vi "AP2_cold_head_control.vi"() -> ()   [LabVIEW 2023]
panel:
  in  "Tab Control":enum32{"Controls", "Monitoring"}(tab)
  in  "stop":bool
  in  "Master Control":bool
  in  "Cold Head Auto Start Time":timestamp format="%<%H:%M:%S>T"
  in  "Target Temperature / K":dbl=4.5 min=4.5 max=500.0 step=1.0
  out "Current Temperature / K":dbl
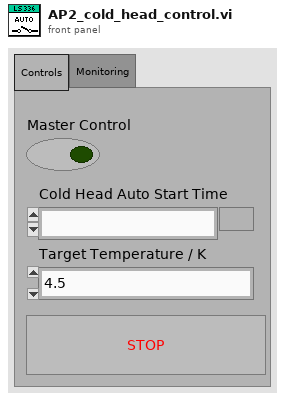
[diagram p1: front panel]
types:
  T1 = cluster{"second":i32, "minute":i32, "hour":i32, "day of month":i32, "month":i32, "year":i32, "day of week":i32, "day of year":i32, "is DST":i32}
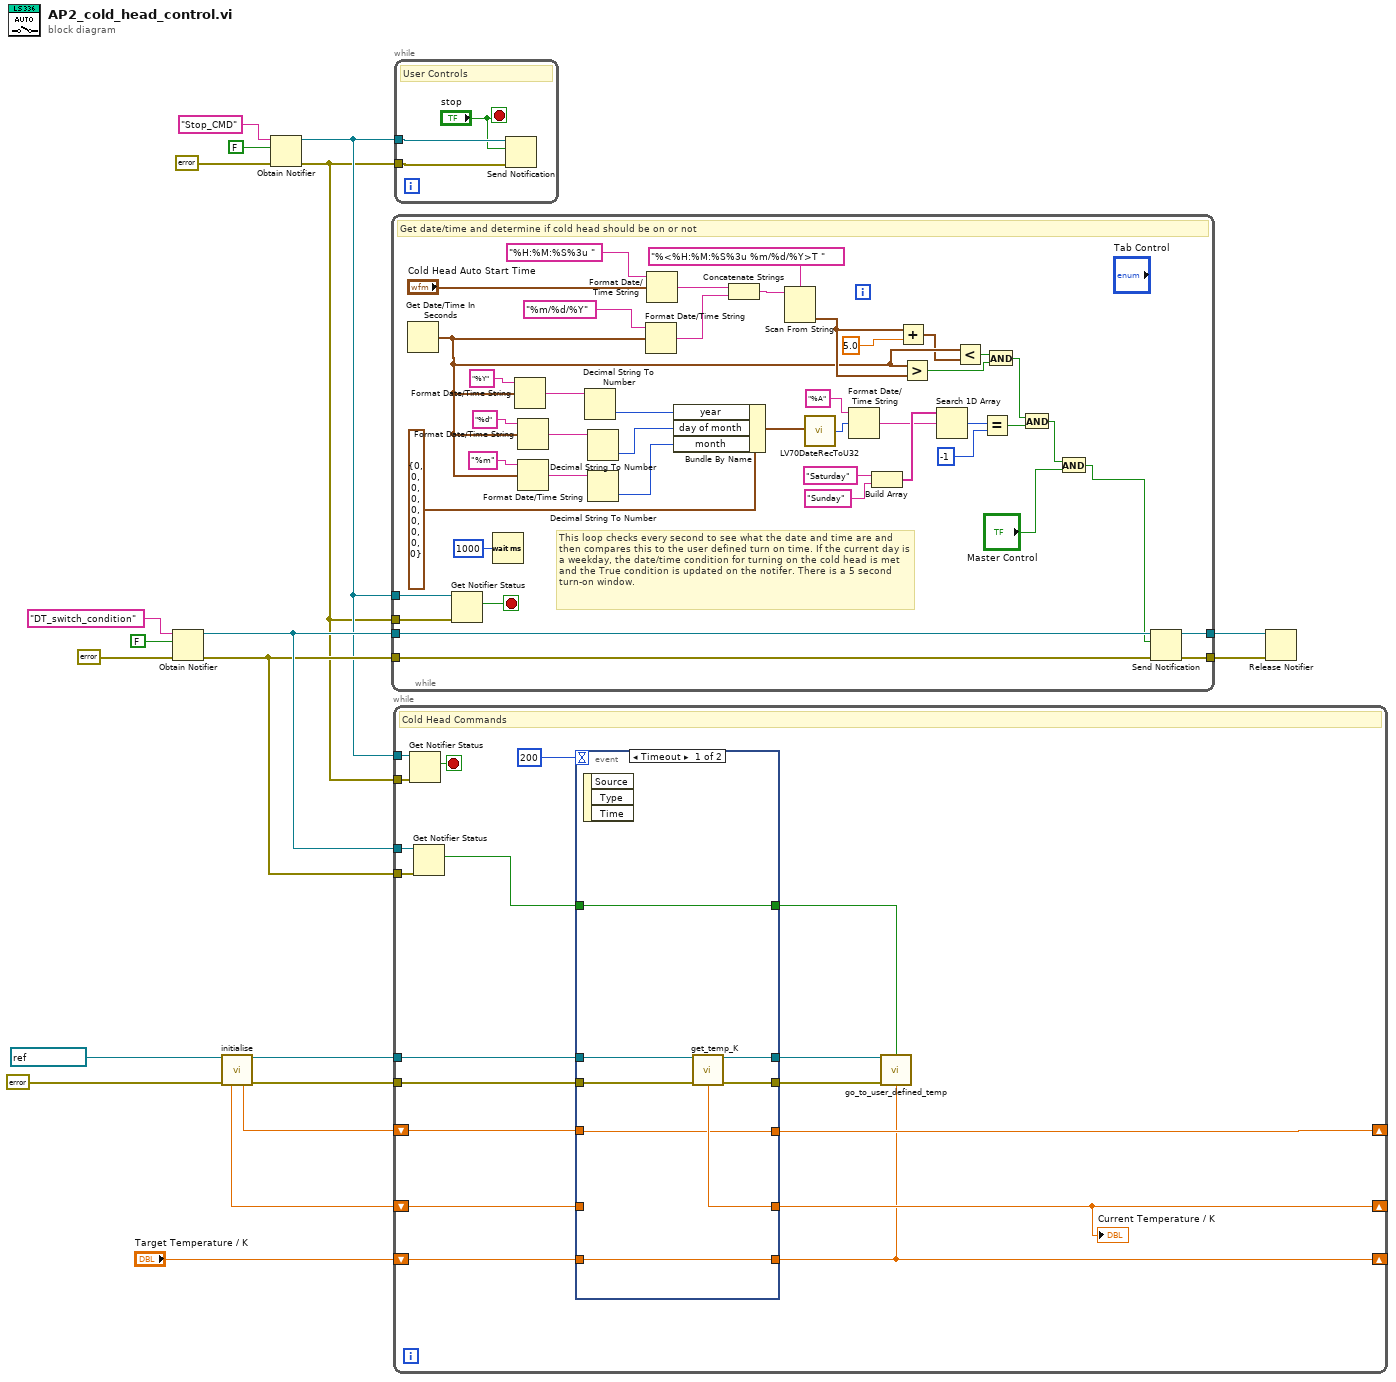
[diagram p0: block diagram]
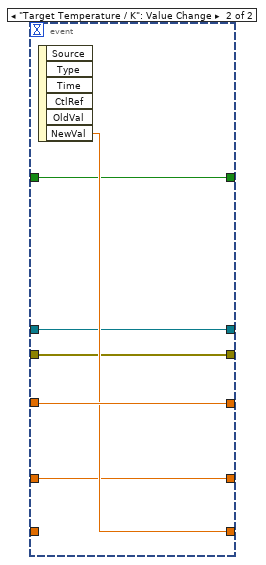
[diagram p2: hidden frame]
diagram:
  n1 = Obtain Notifier(name (unnamed)="DT_switch_condition", notification data type=FALSE, error in (no error)=errorcluster {"status"=FALSE, "code"=0, "source"=""}) -> (notifier out=w14:refnum<notifier>, error out=w13:errorcluster)  [unwired: 1 in, 1 out]
  n2 = call "initialise.vi"("VISA resource name"=refnum<visa-resource-name> "CH_Cntrl", "error in (no error)"=errorcluster {"status"=FALSE, "code"=0, "source"=""}) -> ("VISA resource name out"=w4:refnum<visa-resource-name>, "Cold Head Temperature / K"=w2:dbl, "Current Setpoint / K"=w1:dbl, "error out"=w3:errorcluster)  [unwired: 10 in]
  n3 = Obtain Notifier(name (unnamed)="Stop_CMD", notification data type=FALSE, error in (no error)=errorcluster {"status"=FALSE, "code"=0, "source"=""}) -> (notifier out=w9:refnum<notifier>, error out=w8:errorcluster)  [unwired: 1 in, 1 out]
  n4 = while {
    tunnel: w14 -> [w36]
    tunnel: w13 -> [w35]
    tunnel: [w34] -> w16
    tunnel: [w33] -> w15
    tunnel: w9 -> [w32]
    tunnel: w8 -> [w31]
    stop <- w30 stop-if-true
    # "This loop checks every second to see what the date and time are and then compares this to the user defined turn on time. If the current day is a weekday, the date/time condition for turning on the cold head is met and the True condition is updated on the notifer. There is a 5 second turn-on window."
    # "Get date/time and determine if cold head should be on or not"
    n5 = Get Date/Time In Seconds() -> (seconds since 1Jan1904=w24:timestamp)
    n6 = Get Notifier Status(notifier=w32, error in (no error)=w31) -> (current notification=w30:bool)  [unwired: 4 out]
    n7 = Wait (ms)(milliseconds to wait=u32 1000) -> ()  [unwired: 1 out]
    n8 = Format Date/Time String(time format string (%c)="%Y", seconds (now)=w24) -> (date/time string=w52:string)  [unwired: 1 in]
    n9 = Format Date/Time String(time format string (%c)="%d", seconds (now)=w24) -> (date/time string=w49:string)  [unwired: 1 in]
    n10 = Format Date/Time String(time format string (%c)="%m", seconds (now)=w24) -> (date/time string=w47:string)  [unwired: 1 in]
    n11 = Decimal String To Number(string=w52) -> (number=w51:i32)  [unwired: 2 in, 1 out]
    n12 = Decimal String To Number(string=w49) -> (number=w46:i32)  [unwired: 2 in, 1 out]
    n13 = Decimal String To Number(string=w47) -> (number=w45:i32)  [unwired: 2 in, 1 out]
    n14 = Format Date/Time String(time format string (%c)="%m/%d/%Y", seconds (now)=w24) -> (date/time string=w64:string)  [unwired: 1 in]
    n15 = Format Date/Time String(time format string (%c)="%H:%M:%S%3u ", seconds (now)="Cold Head Auto Start Time") -> (date/time string=w63:string)  [unwired: 1 in]
    n16 = Bundle By Name(cluster=T1 {"second"=0, "minute"=0, "hour"=0, "day of month"=0, "month"=0, "year"=0, "day of week"=0, "day of year"=0, "is DST"=0} ("date time rec"), "year"=w51, "day of month"=w46, "month"=w45) -> (w54:T1)
    n17 = Concatenate Strings(w63, w64) -> (w62:string)
    n18 = Scan From String(format string="%<%H:%M:%S%3u %m/%d/%Y>T ", input string=w62) -> (output 1=w26:timestamp)  [unwired: 3 in, 3 out]
    n19 = call <vilib>:"LV70DateRecToU32.vi"("date time rec"=w54) -> ("Time"=w56:u32)
    n20 = Format Date/Time String(time format string (%c)="%A", seconds (now)=w56) -> (date/time string=w41:string)  [unwired: 1 in]
    n21 = Build Array("Saturday", "Sunday" ("element")) -> (w42:string[])
    n22 = Add(x=w26, y=5.0) -> (x+y=w23:timestamp)
    n23 = Greater?(x=w24, y=w26) -> (0:w21:bool)
    n24 = Search 1D Array(1D array=w42, element=w41) -> (index of element=w40:i32)  [unwired: 1 in]
    n25 = Less?(x=w24, y=w23) -> (x < y?=w22:bool)
    n26 = Equal?(x=w40, y=-1) -> (x = y?=w37:bool)
    n27 = And(x=w22, y=w21) -> (x .and. y?=w20:bool)
    n28 = And(x=w20, y=w37) -> (x .and. y?=w29:bool)
    n29 = And(x=w29, y="Master Control") -> (x .and. y?=w28:bool)
    n30 = Send Notification(notification=w28, notifier=w36, error in (no error)=w35) -> (notifier out=w34:refnum<notifier>, error out=w33:errorcluster)
  }
  n31 = while {
    tunnel: w14 -> [w82]
    tunnel: w13 -> [w81]
    tunnel: w9 -> [w80]
    tunnel: w8 -> [w79]
    shift-right: [w66] -> _
    shift-left: "Target Temperature / K" -> [w75]
    tunnel: w4 -> [w74]
    tunnel: w3 -> [w73]
    shift-right: [w71] -> _
    shift-left: w2 -> [w72]
    shift-right: [w69] -> _
    shift-left: w1 -> [w70]
    stop <- w78 stop-if-true
    # "Cold Head Commands"
    n32 = Get Notifier Status(notifier=w80, error in (no error)=w79) -> (current notification=w78:bool)  [unwired: 4 out]
    n33 = Get Notifier Status(notifier=w82, error in (no error)=w81) -> (current notification=w76:bool)  [unwired: 4 out]
    n34 = event shown="[0] Timeout" {
      selector: _ -> [_ _]
      dyn-events: _ -> [_ _]
      timeout: 200 -> [_ _]
      tunnel: w76 -> [w83 w91]
      tunnel: w75 -> [w90 _]
      tunnel: [w90 w95] -> w66
      tunnel: w74 -> [w89 w94]
      tunnel: [w88 w94] -> w68
      tunnel: [w87 w93] -> w67
      tunnel: w73 -> [w86 w93]
      tunnel: w72 -> [_ w92]
      tunnel: [w85 w92] -> w71
      tunnel: w70 -> [w84 w96]
      tunnel: [w84 w96] -> w69
      tunnel: [w83 w91] -> w65
      event Timeout {
        n35 = event-data() -> ()  [unwired: 1 in, 3 out]
        n36 = call "get_temp_K.vi"("VISA resource name"=w89, "error in (no error)"=w86) -> ("VISA resource name out"=w88:refnum<visa-resource-name>, "Cold Head Temperature / K"=w85:dbl, "error out"=w87:errorcluster)  [unwired: 11 in]
      }
      event "Target Temperature / K": Value Change {
        n37 = event-data() -> ("NewVal"=w95:dbl)  [unwired: 1 in, 5 out]
      }
    }
    "Current Temperature / K" <- w71
    n38 = call "go_to_user_defined_temp.vi"("VISA resource name"=w68, "Status  Control"=w65, "error in (no error)"=w67, "Target Temperature / K"=w66) -> ()  [unwired: 10 in, 2 out]
  }
  n39 = while {
    tunnel: w9 -> [w99]
    tunnel: w8 -> [w98]
    stop <- "stop" stop-if-true
    # "User Controls"
    n40 = Send Notification(notification="stop", notifier=w99, error in (no error)=w98) -> ()  [unwired: 2 out]
  }
  n41 = Release Notifier(notifier=w16, error in (no error)=w15) -> ()  [unwired: 1 in, 3 out]
